vi "PWM Control.vi"() -> ()   [LabVIEW 2019]
uses:
  <vilib>/Utility/error.llb/DialogType.ctl
  <vilib>/DAQmx/write.llb/DAQmx Write (Counter Frequency 1Chan 1Samp).vi
  <vilib>/DAQmx/create/channels.llb/DAQmx Create Channel (CO-Pulse Generation-Frequency).vi
  <vilib>/DAQmx/configure/timing.llb/DAQmx Timing (Implicit).vi
  <vilib>/DAQmx/miscellaneous.llb/DAQmx Fill In Error Info.vi
  <resource>/objmgr/daqmx.rc
panel:
  in  "Liga aquecedor":bool
  in  "stop geral":bool
  in  "Frequency":dbl=1.0 format="%.6f"
  in  "Duty Cycle":dbl=0.225 format="%.6f"
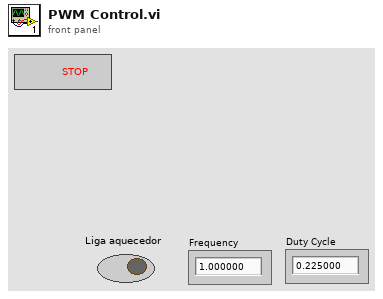
[diagram p1: front panel]
types:
  T1 = typedef "DialogType.ctl" = u16
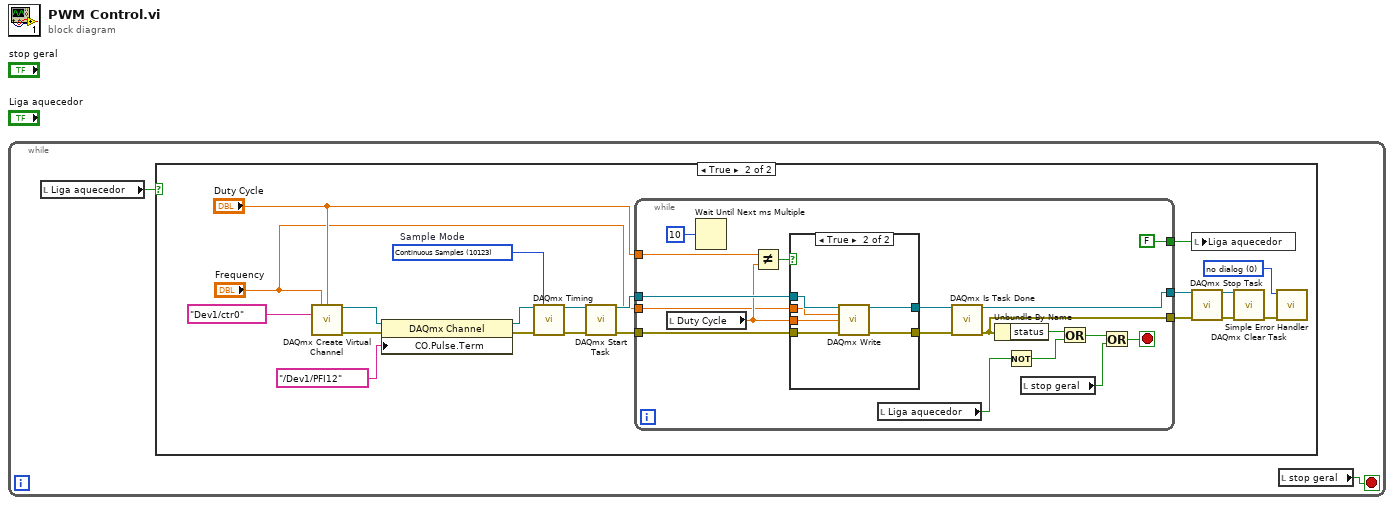
[diagram p0: block diagram]
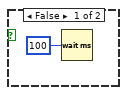
[diagram p2: hidden frame]
diagram:
  n1 = while {
    stop <- w1 stop-if-true
    n2 = local read "Liga aquecedor"() -> (w2:bool)
    n3 = case shown="True" w2 {
      frame False {
        n4 = Wait (ms)(milliseconds to wait=u32 100) -> ()  [unwired: 1 out]
      }
      frame True {
        w8 = T1 0 items=["no dialog", "OK message", "continue or stop message", "OK message + warnings", "continue/stop + warnings"] ("type of dialog (OK msg:1)")
        w19 = 10123 items=["Finite Samples"=10178, "Continuous Samples"=10123, "Hardware Timed Single Point"=12522]  # Sample Mode
        n5 = call-poly <vilib>:"DAQmx Create Virtual Channel.vi"("frequency"="Frequency", "duty cycle"="Duty Cycle", "counter"=tag "Dev1/ctr0" ("Counter")) -> ("task out"=w22:refnum<k21>, "error out"=w21:errorcluster)  [unwired: 11 in]
        n6 = property class="DAQmx Channel"(reference=w22, error in=w21, "CO.Pulse.Term"=tag "/Dev1/PFI12" ("Output Terminal")) -> (reference out=w18:refnum<k21>, error out=w17:errorcluster)
        n7 = call-poly <vilib>:"DAQmx Timing.vi"("task/channels in"=w18, "sample mode"=w19, "error in"=w17) -> ("task out"=w16:refnum<k21>, "error out"=w15:errorcluster)  [unwired: 11 in]
        n8 = call <vilib>:"DAQmx Start Task.vi"("task/channels in"=w16, "error in"=w15) -> ("task out"=w14:refnum<k21>, "error out"=w13:errorcluster)  [unwired: 12 in]
        n9 = while {
          tunnel: w14 -> [w31]
          tunnel: w13 -> [w29]
          tunnel: [w40] -> w10
          tunnel: [w41] -> w11
          tunnel: [FALSE ("Liga aquecedor")] -> w7
          tunnel: "Duty Cycle" -> [w27]
          tunnel: "Frequency" -> [w24]
          stop <- w34 stop-if-true
          n10 = local read "Duty Cycle"() -> (w25:dbl)
          n11 = Wait Until Next ms Multiple(millisecond multiple=u32 10) -> ()  [unwired: 1 out]
          n12 = Not Equal?(x=w27, y=w25) -> (x != y?=w26:bool)
          n13 = case shown="True" w26 {
            tunnel: [w43 w46] -> w30
            tunnel: w31 -> [w43 w47]
            tunnel: [w42 w48] -> w28
            tunnel: w29 -> [w42 w49]
            tunnel: w25 -> [_ w45]
            tunnel: w24 -> [_ w44]
            frame False {
            }
            frame True {
              n14 = call-poly <vilib>:"DAQmx Write.vi"("task/channels in"=w47, "frequency"=w44, "duty cycle"=w45, "error in"=w49) -> ("task out"=w46:refnum<k21>, "error out"=w48:errorcluster)  [unwired: 9 in, 1 out]
            }
          }
          n15 = local read "Liga aquecedor"() -> (w37:bool)
          n16 = call <vilib>:"DAQmx Is Task Done.vi"("task/channels in"=w30, "error in"=w28) -> ("task out"=w41:refnum<k21>, "error out"=w40:errorcluster)  [unwired: 11 in, 1 out]
          n17 = Unbundle By Name(w40) -> ("status"=w39:bool)
          n18 = Not(x=w37) -> (.not. x?=w35:bool)
          n19 = local read "stop geral"() -> (w32:bool)
          n20 = Or(x=w39, y=w35) -> (x .or. y?=w33:bool)
          n21 = Or(x=w33, y=w32) -> (x .or. y?=w34:bool)
        }
        n22 = local write "Liga aquecedor"(w7) -> ()
        n23 = call <vilib>:"DAQmx Stop Task.vi"("task/channels in"=w11, "error in"=w10) -> ("task out"=w6:refnum<k21>, "error out"=w12:errorcluster)  [unwired: 12 in]
        n24 = call <vilib>:"DAQmx Clear Task.vi"("task in"=w6, "error in"=w12) -> ("error out"=w9:errorcluster)  [unwired: 13 in]
        n25 = call <vilib>:"Simple Error Handler.vi"("error code (no error:0)"=w8, "error in (no error)"=w9) -> ()  [unwired: 3 in, 5 out]
      }
    }
    n26 = local read "stop geral"() -> (w1:bool)
  }
